vi "server.vi"() -> ()   [LabVIEW 2019]
uses:
  <vilib>/sound2/lvsound2.llb/Sound Data Format.ctl
  <vilib>/sound2/lvsound2.llb/Sampling Mode.ctl
  <vilib>/sound2/lvsound2.llb/Sound Output Write (DBL Single).vi
panel:
  in  "Volume":dbl
  out "calculated_samples":dbl[](array[numeric])
  out "total_len":dbl
  in  "instrument option":string
  in  "stop looping":bool
  in  "start_looping":bool
  out "frequency_received":dbl
  out "error out":errorcluster
  in  "instrument stop":bool
  in  "sound format":T1={"sample rate (S/s)"=22050.0, "number of channels"=1, "bits per sample"=16}
  out "audio to be looped":waveform(dbl)(graph)
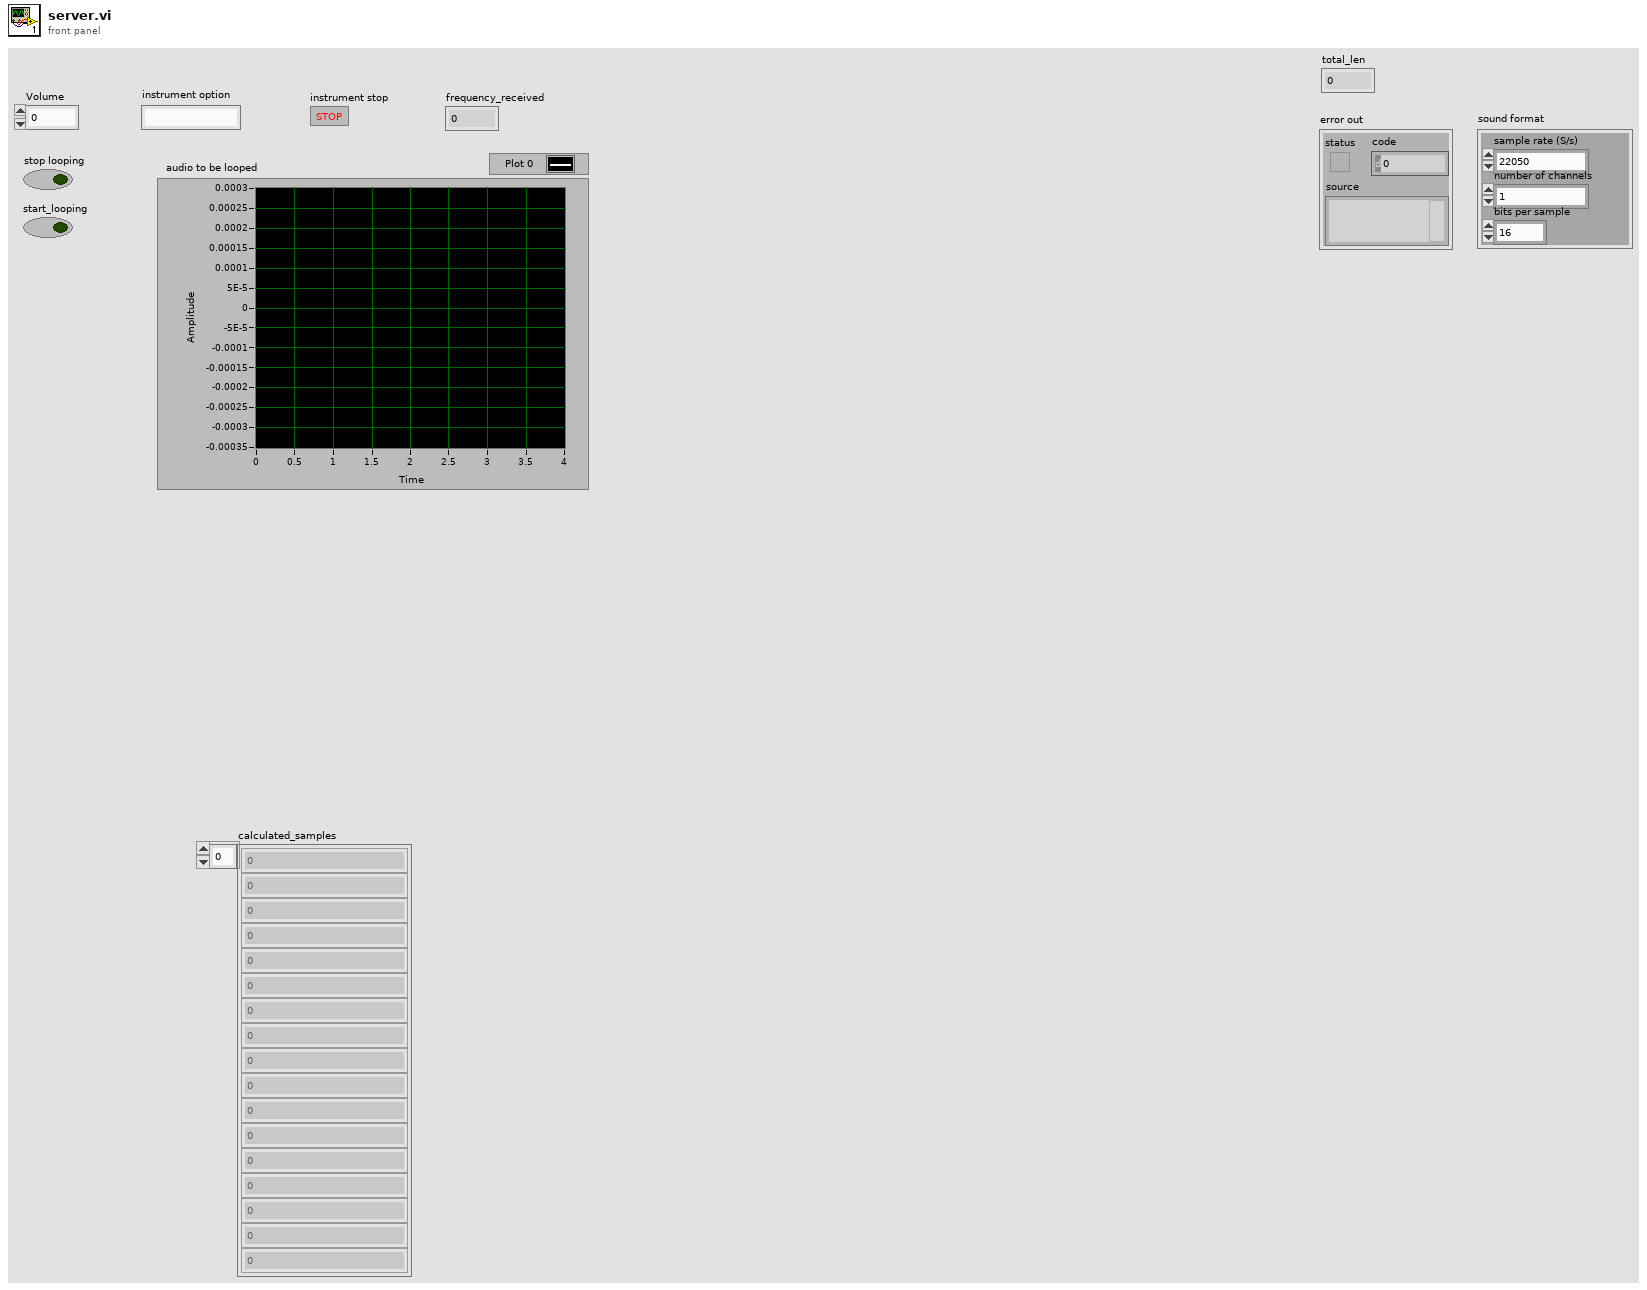
[diagram p1: front panel]
types:
  T1 = typedef "Sound Data Format.ctl" = cluster{"sample rate (S/s)":dbl, "number of channels":i32, "bits per sample":i32}
  T2 = typedef "Sampling Mode.ctl" = i32
  T3 = typedef "Sound Output Task ID.ctl" = u32
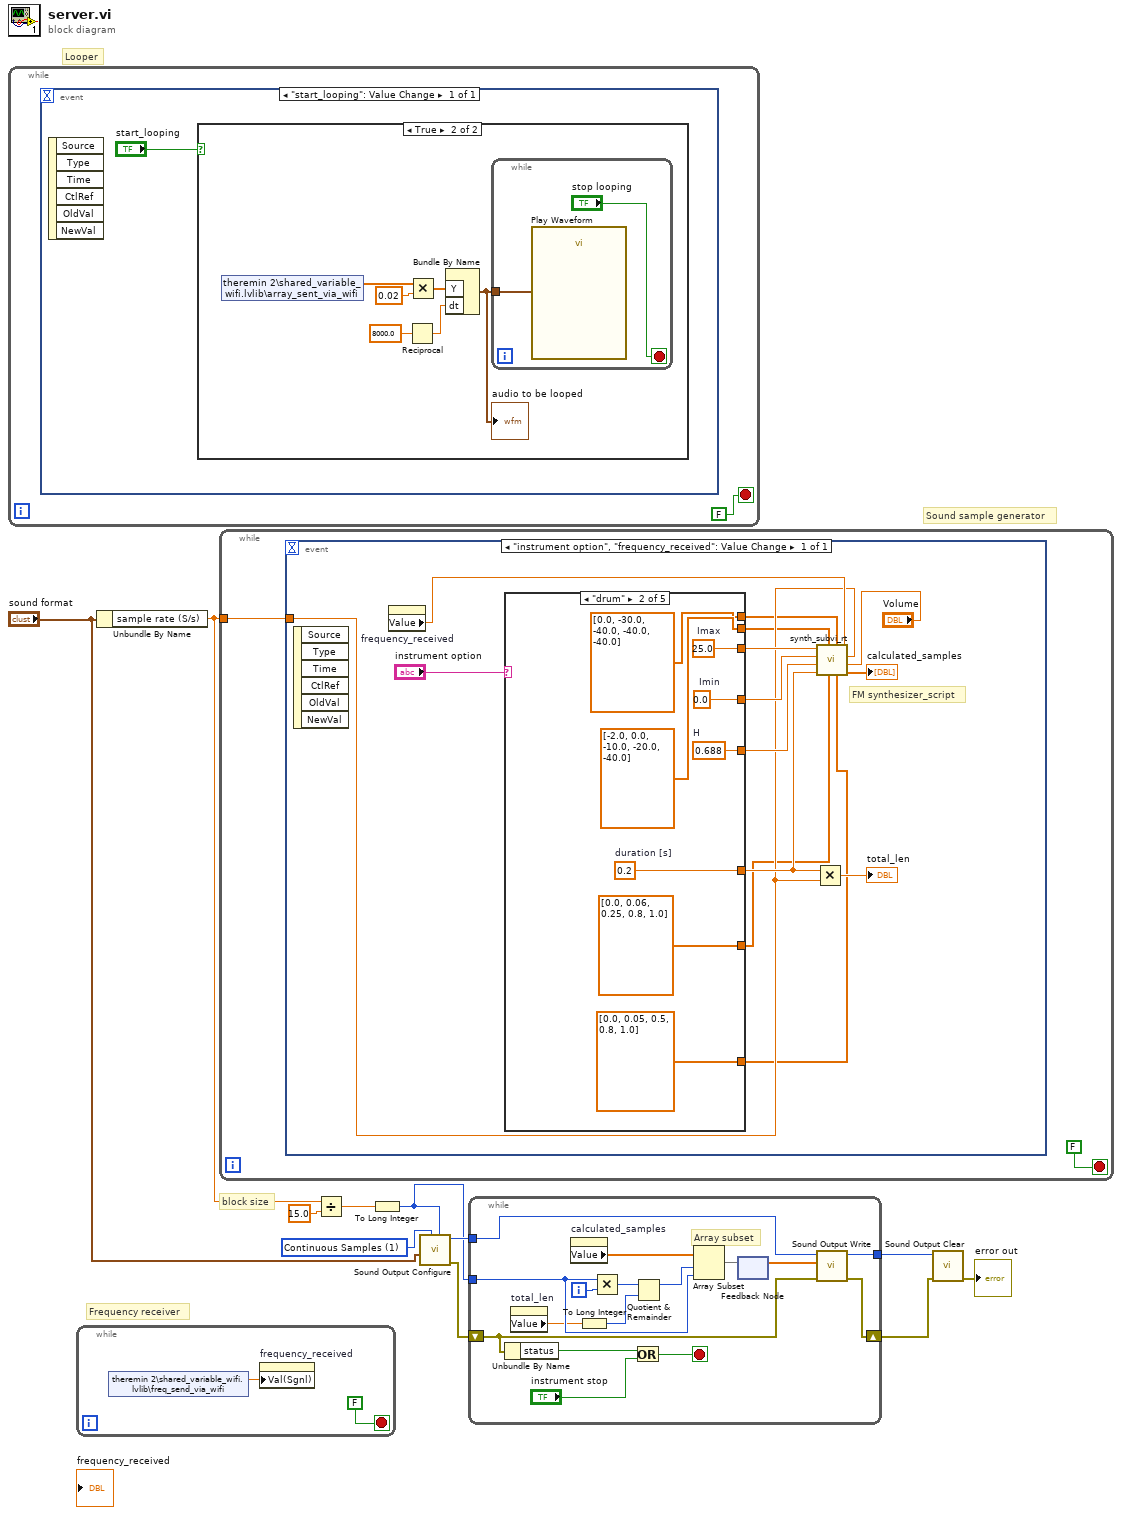
[diagram p0: block diagram]
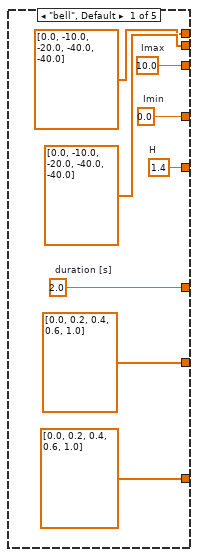
[diagram p3: hidden frame]
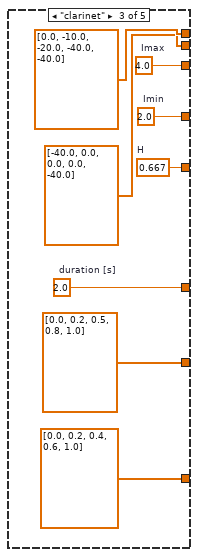
[diagram p4: hidden frame]
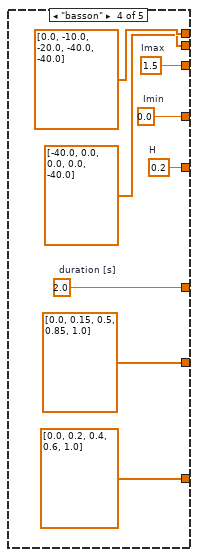
[diagram p5: hidden frame]
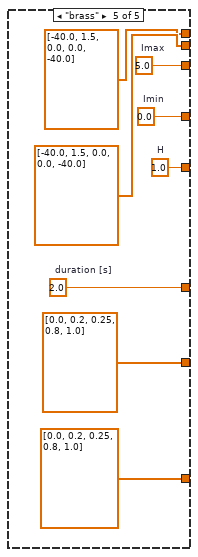
[diagram p6: hidden frame]
diagram:
  w7 = T2 1 items=["Finite Samples", "Continuous Samples"] ("sample mode")
  # "Frequency receiver"
  # "Sound sample generator"
  # "Looper"
  # "block size"
  n1 = while {
    stop <- FALSE stop-if-true
    n2 = event shown="[0] \"start_looping\": Value Change" {
      selector: _ -> [_]
      dyn-events: _ -> [_]
      timeout: _ -> [_]
      event "start_looping": Value Change {
        n3 = event-data() -> ()  [unwired: 1 in, 6 out]
        n4 = case shown="True" "start_looping" {
          frame False {
          }
          frame True {
            n5 = shared-variable "theremin 2\\shared_variable_wifi.lvlib\\array_sent_via_wifi"() -> (w15:dbl[])  [unwired: 1 in, 1 out]
            n6 = Reciprocal(x=8000.0) -> (1/x=w18:dbl)
            n7 = Multiply(x=w15, y=0.02) -> (x*y=w16:dbl[])
            n8 = Bundle By Name("Y"=w16, "dt"=w18) -> (w19:waveform(dbl))  [unwired: 1 in]
            "audio to be looped" <- w19
            n9 = while {
              tunnel: w19 -> [w21]
              stop <- "stop looping" stop-if-true
              n10 = call "Play Waveform"("Data"=w21) -> ()  [unwired: 18 in, 1 out]
            }
          }
        }
      }
    }
  }
  n11 = while {
    stop <- FALSE stop-if-true
    n12 = shared-variable "theremin 2\\shared_variable_wifi.lvlib\\freq_send_via_wifi"() -> (w23:dbl)  [unwired: 1 in, 1 out]
    n13 = property on="frequency_received" class="DigNum (strict)"("Val(Sgnl)"=w23) -> ()  [unwired: 2 in, 2 out]
  }
  n14 = Unbundle By Name("sound format") -> ("sample rate (S/s)"=w3:dbl)
  n15 = while {
    tunnel: w3 -> [w25]
    stop <- FALSE stop-if-true
    n16 = event shown="[0] \"instrument option\", \"frequency_received\": Value Change" {
      selector: _ -> [_]
      dyn-events: _ -> [_]
      timeout: _ -> [_]
      tunnel: w25 -> [w30]
      event "instrument option", "frequency_received": Value Change {
        # "FM synthesizer_script"
        n17 = event-data() -> ()  [unwired: 1 in, 6 out]
        n18 = property on="frequency_received" class="DigNum (strict)"() -> ("Value"=w31:dbl)  [unwired: 2 in, 2 out]
        n19 = case shown="\"drum\"" "instrument option" {
          tunnel: [w47 w51 w63 w64 w79] -> w36
          tunnel: [w46 w50 w62 w65 w78] -> w35
          tunnel: [w45 w49 w56 w66 w77] -> w34
          tunnel: [w44 w48 w57 w67 w76] -> w32
          tunnel: [dbl[] [0.0, -10.0, -20.0, -40.0, -40.0] ("w2(t)") dbl[] [-2.0, 0.0, -10.0, -20.0, -40.0] ("w2(t)") dbl[] [-40.0, 0.0, 0.0, 0.0, -40.0] ("w2(t)") dbl[] [-40.0, 0.0, 0.0, 0.0, -40.0] ("w2(t)") dbl[] [-40.0, 1.5, 0.0, 0.0, -40.0] ("w1(t)")] -> w29
          tunnel: [dbl[] [0.0, -10.0, -20.0, -40.0, -40.0] ("w1(t)") dbl[] [0.0, -30.0, -40.0, -40.0, -40.0] ("w1(t)") dbl[] [0.0, -10.0, -20.0, -40.0, -40.0] ("w1(t)") dbl[] [0.0, -10.0, -20.0, -40.0, -40.0] ("w1(t)") dbl[] [-40.0, 1.5, 0.0, 0.0, -40.0] ("w2(t)")] -> w28
          tunnel: [dbl[] [0.0, 0.2, 0.4, 0.6, 1.0] ("time1") dbl[] [0.0, 0.06, 0.25, 0.8, 1.0] ("time1") dbl[] [0.0, 0.2, 0.5, 0.8, 1.0] ("time1") dbl[] [0.0, 0.15, 0.5, 0.85, 1.0] ("time1") dbl[] [0.0, 0.2, 0.25, 0.8, 1.0] ("time1")] -> w27
          tunnel: [dbl[] [0.0, 0.2, 0.4, 0.6, 1.0] ("time2") dbl[] [0.0, 0.05, 0.5, 0.8, 1.0] ("time2") dbl[] [0.0, 0.2, 0.4, 0.6, 1.0] ("time2") dbl[] [0.0, 0.2, 0.4, 0.6, 1.0] ("time2") dbl[] [0.0, 0.2, 0.25, 0.8, 1.0] ("time2")] -> w26
          frame "bell", Default {
            w44 = 2.0  # duration [s]
            w45 = 1.4  # H
            w46 = 0.0  # Imin
            w47 = 10.0  # Imax
          }
          frame "drum" {
            w48 = 0.2  # duration [s]
            w49 = 0.688  # H
            w50 = 0.0  # Imin
            w51 = 25.0  # Imax
          }
          frame "clarinet" {
            w57 = 2.0  # duration [s]
            w56 = 0.667  # H
            w62 = 2.0  # Imin
            w63 = 4.0  # Imax
          }
          frame "basson" {
            w67 = 2.0  # duration [s]
            w66 = 0.2  # H
            w65 = 0.0  # Imin
            w64 = 1.5  # Imax
          }
          frame "brass" {
            w76 = 2.0  # duration [s]
            w77 = 1.0  # H
            w78 = 0.0  # Imin
            w79 = 5.0  # Imax
          }
        }
        n20 = Multiply(x=w32, y=w30) -> (x*y=→"total_len":dbl)
        n21 = call "synth_subvi_rt.vi"("A"="Volume", "fs [Hz]"=w30, "fc [Hz]"=w31, "time2"=w26, "w2(t)"=w28, "time1"=w27, "w1(t)"=w29, "duration [s]"=w32, "H"=w34, "Imin"=w35, "Imax"=w36) -> ("discrete_sample"=→"calculated_samples":dbl[])
      }
    }
  }
  n22 = Divide(x=w3, y=15.0) -> (x/y=w5:dbl)
  n23 = To Long Integer(number=w5) -> (32bit integer=w4:i32)
  n24 = call <vilib>:"Sound Output Configure.vi"("number of samples/ch"=w4, "sample mode"=w7, "sound format"="sound format") -> ("error out"=w10:errorcluster, "task ID"=w8:T3)  [unwired: 7 in]
  n25 = while {
    tunnel: w8 -> [w94]
    tunnel: [w89] -> w1
    shift-right: [w95] -> w9
    shift-left: w10 -> [w93]
    tunnel: w4 -> [w85]
    i -> [w88]
    stop <- w90 stop-if-true
    # "Array subset"
    n26 = Unbundle By Name(w93) -> ("status"=w91:bool)
    n27 = property on="total_len" class="DigNum (strict)"() -> ("Value"=w80:dbl)  [unwired: 2 in, 2 out]
    n28 = property on="calculated_samples" class="Arr (strict)"() -> ("Value"=w81:dbl[])  [unwired: 2 in, 2 out]
    n29 = To Long Integer(number=w80) -> (32bit integer=w82:i32)
    n30 = Multiply(x=w85, y=w88) -> (x*y=w84:i32)
    n31 = Or(x=w91, y="instrument stop") -> (x .or. y?=w90:bool)
    n32 = Quotient & Remainder(x=w84, y=w82) -> (x-y*floor(x/y)=w83:i32)  [unwired: 1 out]
    n33 = Array Subset(array=w81, index=w83, length=w85) -> (w87:dbl[])
    n34 = feedback-in #1(w87) -> ()
    n35 = feedback #1() -> (w86:dbl[])  [unwired: 1 in]
    n36 = call-poly <vilib>:"Sound Output Write.vi"("error in (no error)"=w93, "data"=w86, "task ID"=w94) -> ("error out"=w95:errorcluster, "task ID out"=w89:T3)  [unwired: 7 in]
  }
  n37 = call <vilib>:"Sound Output Clear.vi"("error in (no error)"=w9, "task ID"=w1) -> ("error out"=→"error out":errorcluster)  [unwired: 9 in]
